vi "Transmitter.vi"(8 "ErrorArray":errorcluster[](array[cluster]), 9 "XMLData":string, 10 "Command":string) -> (0 "ErrorArray":errorcluster[](array[cluster]), 2 "xml string":string)   [LabVIEW 2017, in "Comms.lvlib"]
uses:
  Comms.lvlib
  CommsData.ctl
  <userlib>/NIST/Socket Class/Classes/Socket.TCP/Socket.TCP.lvclass
  <userlib>/NIST/NISTErrorLib/NISTErrorLib.lvlib
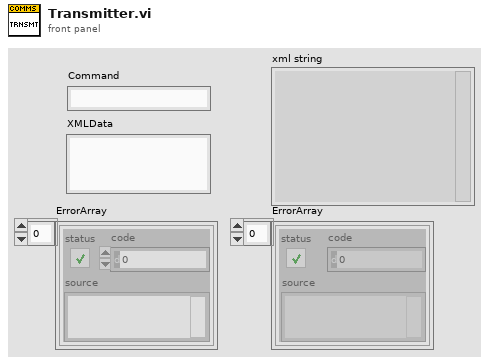
[diagram p1: front panel]
types:
  T1 = typedef "Comms.lvlib/CommsData.ctl" = cluster{"Command":string, "XMLData":string}
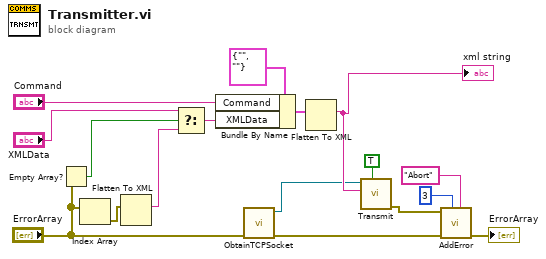
[diagram p0: block diagram]
diagram:
  n1 = Empty Array?(array="ErrorArray") -> (empty?=w1:bool)
  n2 = Index Array(array="ErrorArray") -> (element=w4:errorcluster)  [unwired: 1 in]
  n3 = Flatten To XML(anything=w4) -> (xml string=w3:string)
  n4 = Select(t="XMLData", s=w1, f=w3) -> (s? t:f=w2:string)
  n5 = Bundle By Name(cluster=T1 {"Command"="", "XMLData"=""} ("CommsData"), "Command"="Command", "XMLData"=w2) -> (w12:T1)
  n6 = call "ObtainTCPSocket.vi"("ErrorArray"="ErrorArray") -> ("ErrorArray"=w9:errorcluster[], "SocketRef"=w14:refnum<class "Socket.TCP.lvclass">)  [unwired: 9 in]
  n7 = Flatten To XML(anything=w12) -> (xml string=w15:string)
  "xml string" <- w15
  n8 = call-dynamic "Transmit.vi"("packet? (f)"=TRUE, "data"=w15, "Socket.TCP in"=w14) -> ("error out"=w10:errorcluster)  [unwired: 6 in, 2 out]
  n9 = call <userlib>:"AddError.vi"("Severity"="Abort", "Priority"=u8 3, "ErrorArray"=w9, "error in (no error)"=w10) -> ("ErrorArray"=→"ErrorArray":errorcluster[])  [unwired: 6 in, 1 out]
